vi "Write Attributes Metadata.vi"(10 "Attributes Metadata":refnum<class "Attributes Metadata.lvclass">, 11 "Attributes in":refnum<class "Attributes.lvclass">) -> (3 "Attributes out":refnum<class "Attributes.lvclass">)   [LabVIEW 2020, in "jettl.lvlib" / "Attributes.lvclass"]
uses:
  Attributes.lvclass
  Attributes Metadata/Attributes Metadata.lvclass
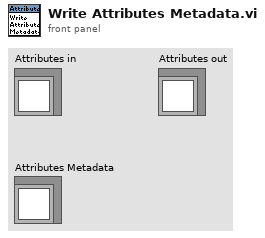
[diagram p1: front panel]
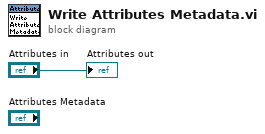
[diagram p0: block diagram]
diagram:
  "Attributes out" <- "Attributes in"
